vi "GetTerms3.vi"(0 "XRef":T10, 1 "State In":T9) -> (14 "Terms":T1)   [LabVIEW 2012, in "IsA.xnode"]
doc: "This ability VI is used to describe your terminals to LabVIEW. Terms is an array of clusters describing the XNode's terminals.\n ID: A unique string identifying the terminal.\n Name: The name of the terminal visible to the user. Remember to localize it.\n Type: The data type of the terminal (as a Variant). The data put in the variant will be used as the default for the input terminal if it's left unwired.\n Bounds: A rectangle defining the bounds of the terminal relative to the bounds of the XNode. The bounds must be within the bounds of the XNode, and for whiskers to draw properly, they must be flush with at least one side of the XNode.\n Input?: Indicates whether or not this terminals is an input.\n Required?: Indicates whether the user must wire this terminal for the XNode to not be broken. Ignored on outputs.\n Recommended?: Indicates whether the terminal is recommended.\n Hidden?: Indicates whether the terminal is hidden. When a terminal is hidden, it cannot be wired to via user interaction or scripting. However, if it is already wired to when the hidden flag is changed to true, it will remain wired.\n Adaptive?: Indicates that the term should change to match the type of its source if it is wired.\n Direction?: Indicates what direction the wire stub should point. Choose auto to let LV decide based on the terms bounds being on the nodes edge.\n \n The IDs are used by LabVIEW to keep track of your terminals. When you respecify your terminals, LabVIEW can tell whther terminals are new, deleted, or moved by the unique IDs. The order is irrelevant. If you move a terminal, then any wire connected to it will move with it.\n \n If you want to update your terminals, you should return the UpdateTerms reply in one of your ability VIs.\n\nDefault behavior: None.\n\nThis ability does not provide UI and OS messages are not handled."
uses:
  IsA.xnode
  <vilib>/XNodeSupport/XNodeXNodeRef.ctl
  State.ctl
  <vilib>/XNodeSupport/XNodeTerm3Array.ctl
  <vilib>/XNodeSupport/XNodeTerm3.ctl
  <vilib>/XNodeSupport/XNodeString.ctl
  <vilib>/XNodeSupport/XNodeVariant.ctl
  <vilib>/XNodeSupport/XNodeRect32.ctl
  <vilib>/XNodeSupport/XNodeInt.ctl
  <vilib>/XNodeSupport/XNodeBool.ctl
  <vilib>/XNodeSupport/XNodeTermDirection.ctl
  <vilib>/XNodeSupport/NI_XNodeSupport.lvlib
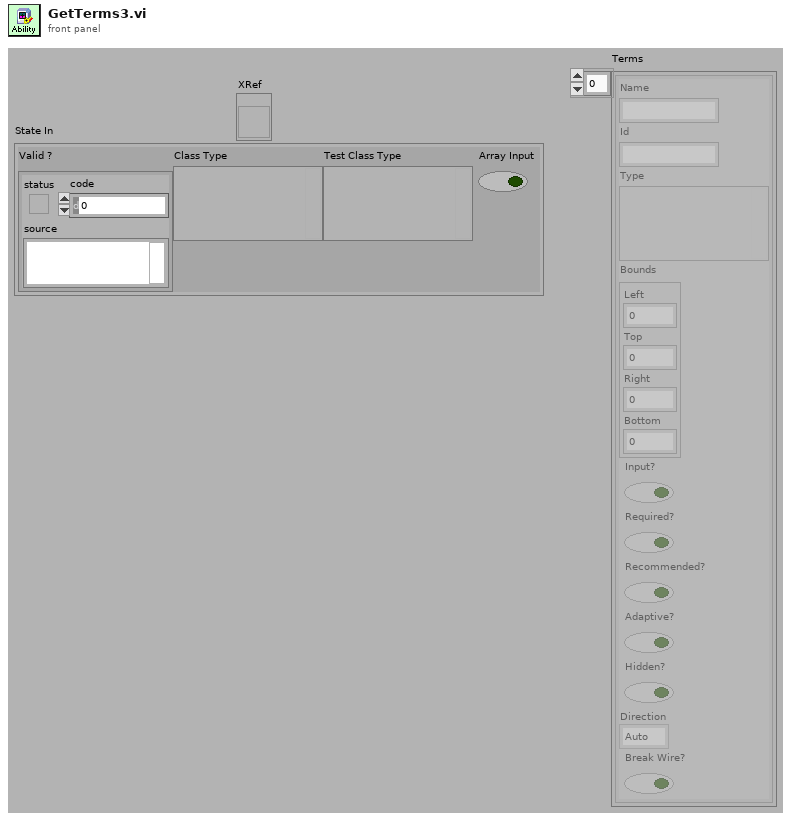
[diagram p1: front panel]
types:
  T1 = typedef "NI_XNodeSupport.lvlib/XNodeTerm3Array.ctl" = T2[]
  T2 = typedef "NI_XNodeSupport.lvlib/XNodeTerm3.ctl" = cluster{"Name":T3, "Id":T3, "Type":T4, "Bounds":T5, "Input?":T7, "Required?":T7, "Recommended?":T7, "Adaptive?":T7, "Hidden?":T7, "Direction":T8, "Break Wire?":T7}
  T3 = typedef "NI_XNodeSupport.lvlib/XNodeString.ctl" = string
  T4 = typedef "NI_XNodeSupport.lvlib/XNodeVariant.ctl" = variant
  T5 = typedef "NI_XNodeSupport.lvlib/XNodeRect32.ctl" = cluster{"Left":T6, "Top":T6, "Right":T6, "Bottom":T6}
  T6 = typedef "NI_XNodeSupport.lvlib/XNodeInt.ctl" = i32
  T7 = typedef "NI_XNodeSupport.lvlib/XNodeBool.ctl" = bool
  T8 = typedef "NI_XNodeSupport.lvlib/XNodeTermDirection.ctl" = enum32{"Auto", "Up", "Down", "Left", "Right", "Center"}
  T9 = typedef "IsA.xnode/State.ctl" = cluster{"Valid ?":errorcluster, "Class Type":variant, "Test Class Type":variant, "Array Input":bool}
  T10 = typedef "NI_XNodeSupport.lvlib/XNodeXNodeRef.ctl" = refnum<vi>
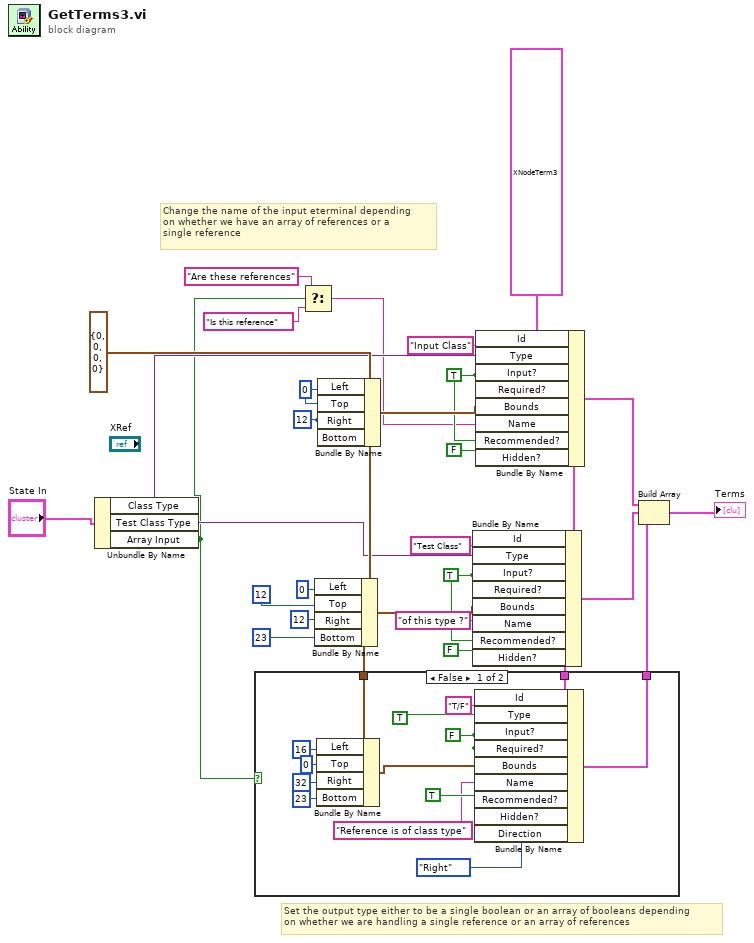
[diagram p0: block diagram]
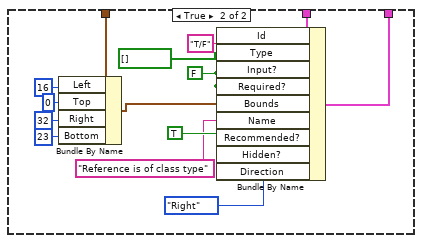
[diagram p2: hidden frame]
diagram:
  w6 = T2 {"Name"="", "Id"="", "Type"=variant, "Bounds"={"Left"=0, "Top"=0, "Right"=0, "Bottom"=0}, "Input?"=FALSE, "Required?"=FALSE, "Recommended?"=FALSE, "Adaptive?"=FALSE, "Hidden?"=FALSE, "Direction"=enum."Left", "Break Wire?"=FALSE} ("Term 3")
  w15 = T6 12 ("Right")
  w16 = T6 0 ("Left")
  w18 = T7 TRUE ("Input?")
  w21 = T7 TRUE ("Input?")
  w28 = T5 {"Left"=0, "Top"=0, "Right"=0, "Bottom"=0} ("Bounds")
  # "Set the output type either to be a single boolean or an array of booleans depending\non whether we are handling a single reference or an array of references"
  # "Change the name of the input eterminal depending\non whether we have an array of references or a\nsingle reference"
  n1 = Unbundle By Name("State In") -> ("Class Type"=w25:variant, "Test Class Type"=w24:variant, "Array Input"=w2:bool)
  n2 = case shown="False" w2 {
    tunnel: w6 -> [w42 w56]
    tunnel: w28 -> [w41 w55]
    tunnel: [w30 w45] -> w8
    frame False {
      w37 = T7 FALSE ("Input?")
      n3 = Bundle By Name(cluster=w41, "Left"=T6 16, "Top"=T6 0, "Right"=T6 32, "Bottom"=T6 23) -> (w40:T5)
      n4 = Bundle By Name(cluster=w42, "Id"=T3 "T/F", "Type"=TRUE, "Input?"=w37, "Required?"=w37, "Bounds"=w40, "Name"=T3 "Reference is of class type", "Recommended?"=TRUE, "Hidden?"=w37, "Direction"=XNodeTermDirection."Right") -> (w30:T2)
    }
    frame True {
      w52 = T7 FALSE ("Input?")
      n5 = Bundle By Name(cluster=w55, "Left"=T6 16, "Top"=T6 0, "Right"=T6 32, "Bottom"=T6 23) -> (w54:T5)
      n6 = Bundle By Name(cluster=w56, "Id"=T3 "T/F", "Type"=bool[] [], "Input?"=w52, "Required?"=w52, "Bounds"=w54, "Name"=T3 "Reference is of class type", "Recommended?"=TRUE, "Hidden?"=w52, "Direction"=XNodeTermDirection."Right") -> (w45:T2)
    }
  }
  n7 = Select(t=T3 "Are these references" ("Name"), s=w2, f=T3 "Is this reference" ("Name")) -> (s? t:f=w1:T3)
  n8 = Bundle By Name(cluster=w28, "Left"=T6 0, "Top"=T6 12, "Right"=T6 12, "Bottom"=T6 23) -> (w26:T5)
  n9 = Bundle By Name(cluster=w28, "Left"=w16, "Top"=w16, "Right"=w15, "Bottom"=w15) -> (w27:T5)
  n10 = Bundle By Name(cluster=w6, "Id"=T3 "Test Class", "Type"=w24, "Input?"=w18, "Required?"=w18, "Bounds"=w26, "Name"=T3 "of this type ?", "Recommended?"=w18, "Hidden?"=T7 FALSE) -> (w9:T2)
  n11 = Bundle By Name(cluster=w6, "Id"=T3 "Input Class", "Type"=w25, "Input?"=w21, "Required?"=w21, "Bounds"=w27, "Name"=w1, "Recommended?"=w21, "Hidden?"=T7 FALSE) -> (w10:T2)
  n12 = Build Array(w10, w9, w8) -> (→"Terms":T2[])
